vi "齿条扭矩电机.vi"() -> ()   [LabVIEW 2013]
panel:
  in  "Change Velocity":dbl=30.0
  out "位置":dbl
  in  "Distance":dbl
  in  "使能":bool
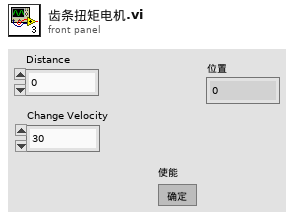
[diagram p1: front panel]
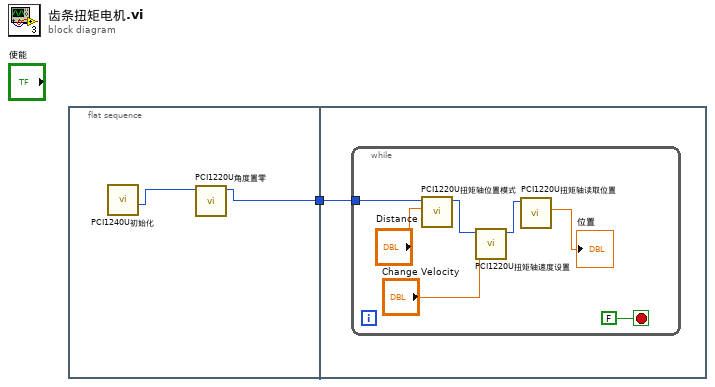
[diagram p0: block diagram]
diagram:
  n1 = flat-sequence {
    tunnel: [w3] -> w1
    tunnel: w1 -> [w4]
    frame #0 {
      n2 = call "PCI1240U初始化.vi"() -> ("旋转电机"=w2:u32)  [unwired: 6 in, 5 out]
      n3 = call "PCI1220U角度置零.vi"("AxisHandle IN"=w2) -> ("AxisHandle OUT"=w3:u32)  [unwired: 10 in]
    }
    frame #1 {
      n4 = while {
        tunnel: w4 -> [w8]
        stop <- FALSE stop-if-true
        n5 = call "PCI1220U扭矩轴位置模式.vi"("Distance"="Distance", "AxisHandle IN"=w8) -> ("AxisHandle OUT"=w7:u32)  [unwired: 8 in, 1 out]
        n6 = call "PCI1220U扭矩轴速度设置.vi"("Change Velocity"="Change Velocity", "AxisHandle IN"=w7) -> ("AxisHandle OUT"=w6:u32)  [unwired: 9 in]
        n7 = call "PCI1220U扭矩轴读取位置.vi"("AxisHandle IN"=w6) -> ("位置"=→"位置":dbl)  [unwired: 9 in, 1 out]
      }
    }
  }
